vi "nirviEmuArrayToTypes_template.vi"(0 "type":bool, 2 "variant":bool) -> (1 "element":bool)   [LabVIEW 2017]
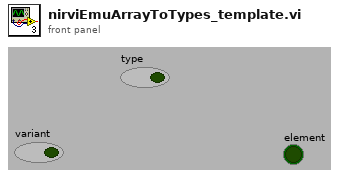
[diagram p1: front panel]
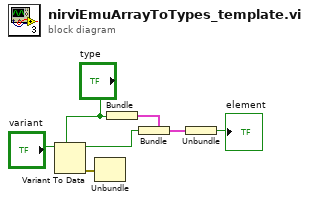
[diagram p0: block diagram]
diagram:
  n1 = Variant To Data(type="type", Variant="variant") -> (data=w3:bool, error out=w7:errorcluster)  [unwired: 1 in]
  n2 = Unbundle(w7) -> ()  [unwired: 3 out]
  n3 = Bundle("type"="type") -> (w5:cluster{"type":bool})  [unwired: 1 in]
  n4 = Bundle(cluster=w5, "type"=w3) -> (w4:cluster{"type":bool})
  n5 = Unbundle(w4) -> ("type"=→"element":bool)
